vi "from_string.vi"(8 "error in (no error)":errorcluster, 10 "toml":string) -> (0 "error out":errorcluster, 3 "Doc out":refnum<class "Doc.lvclass">)   [LabVIEW 2020, in "toml_edit.lvlib" / "Doc.lvclass"]
uses:
  Doc.lvclass
  Doc.lvclass/Doc.ctl
  dragon_toml_64.dll
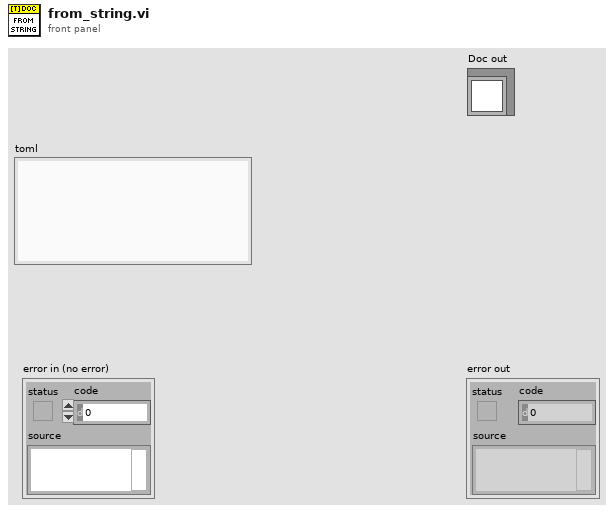
[diagram p1: front panel]
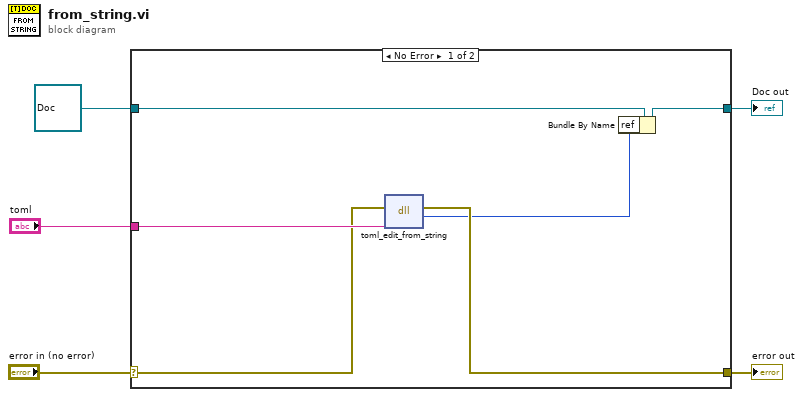
[diagram p0: block diagram]
diagram:
  n1 = case shown="No Error" "error in (no error)" {
    selector: "error in (no error)" -> [w9 w13]
    tunnel: [w8 w13] -> w4
    tunnel: [w7 w12] -> w2
    tunnel: refnum<class "Doc.lvclass"> refnum ("Doc in") -> [w11 w12]
    tunnel: "toml" -> [w10 _]
    frame No Error {
      n2 = dll-call lib="C:/Projects/labview-project-load-tools/rust_src/toml_edit_dll/lv_src/dragon_toml_*.dll" fn="toml_edit_from_string"(error in=w9, "toml_string"=w10) -> (error out=w8:errorcluster, "doc"=w6:u64)  [unwired: 3 in, 1 out]
      n3 = Bundle By Name(cluster=w11, "ref"=w6) -> (w7:refnum<class "Doc.lvclass">)
    }
    frame Error {
    }
  }
  "error out" <- w4
  "Doc out" <- w2
